vi "RampParaToString_calc.vi"(0 "#Points":u32, 1 "Mode":T1(ring), 3 "RampParameter":dbl[](array[numeric])=[0.0, 30.0, 1.0, 20.0] format="%.2f", 4 "Maximum Allowed Current":dbl=100.0 format="%.2f") -> (5 "Output String":string, 6 "#Points output":u32, 7 "Field Step":dbl=0.5 format="%.2f")   [LabVIEW 2021]
doc: "This Vi extract current field and set the scan continue boolean variable.\n\nThe field step can be either positive or negative.\n\nIf any of the absolute field value exceeds the maximum allowed limit, it will be replaced with the maximum field value itself"
panel:
  out "Field Array List":dbl[](array[numeric])=[0.0, 0.5, 1.0, 1.5, 2.0, 2.5, 3.0, 3.5, 4.0, 4.5, 5.0, 5.5, 6.0, 6.5, 7.0, 7.5, 8.0, 8.5, 9.0, 9.5, 10.0, 10.5, 11.0, 11.5, 12.0, 12.5, 13.0, 13.5, 14.0, 14.5, 15.0, 15.5, 16.0, 16.5, 17.0, 17.5, 18.0, 18.5, 19.0, 19.5, 20.0, 20.5, 21.0, 21.5, 22.0, 22.5, 23.0, 23.5, 24.0, 24.5, 25.0, 25.5, 26.0, 26.5, 27.0, 27.5, 28.0, 28.5, 29.0, 29.5, 30.0, 30.5, 31.0, 31.5, 32.0, 32.5, 33.0, 33.5, 34.0, 34.5, 35.0, 35.5, 36.0, 36.5, 37.0, 37.5, 38.0, 38.5, 39.0, 39.5, 40.0, 40.5, 41.0, 41.5, 42.0, 42.5, 43.0, 43.5, 44.0, 44.5]
  out "Final Field":dbl=45.0 format="%.2f"
  out "Initial Field":dbl format="%.2f"
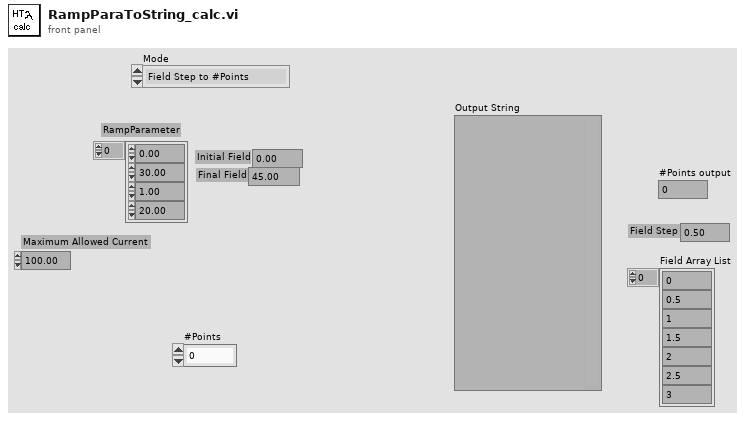
[diagram p1: front panel]
types:
  T1 = enum8{"Field Step to #Points", "#Points to Field Steps"}
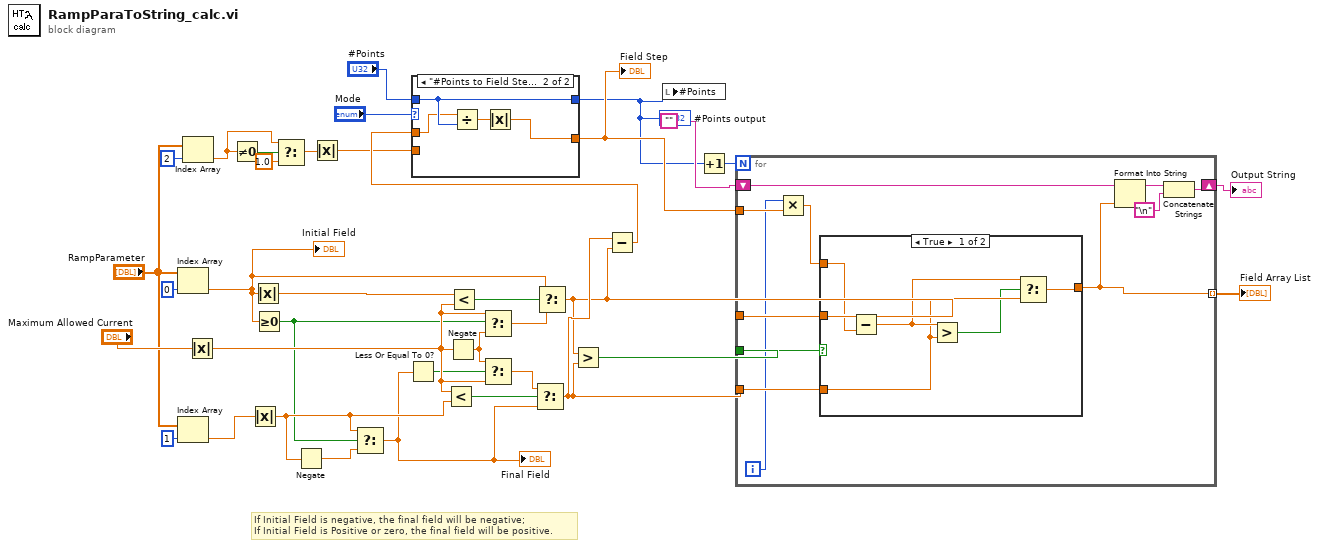
[diagram p0: block diagram]
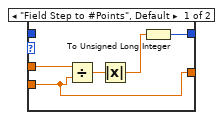
[diagram p2: hidden frame]
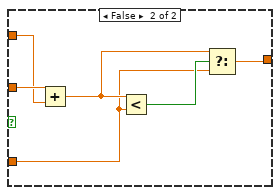
[diagram p3: hidden frame]
diagram:
  # "If Initial Field is negative, the final field will be negative;\nIf Initial Field is Positive or zero, the final field will be positive."
  n1 = Index Array(array="RampParameter", index=0) -> (element=w32:dbl)
  "Initial Field" <- w32
  n2 = Index Array(array="RampParameter", index=1) -> (element=w31:dbl)
  n3 = Index Array(array="RampParameter", index=2) -> (element=w9:dbl)
  n4 = Absolute Value(x="Maximum Allowed Current") -> (abs(x)=w35:dbl)
  n5 = Not Equal To 0?(x=w9) -> (x != 0?=w10:bool)
  n6 = Absolute Value(x=w31) -> (abs(x)=w16:dbl)
  n7 = Absolute Value(x=w32) -> (abs(x)=w36:dbl)
  n8 = Greater Or Equal To 0?(x=w32) -> (x >= 0?=w15:bool)
  n9 = Select(t=w9, s=w10, f=1.0) -> (s? t:f=w4:dbl)
  n10 = Negate(x=w16) -> (-x=w14:dbl)
  n11 = Absolute Value(x=w4) -> (abs(x)=w2:dbl)
  n12 = Select(t=w16, s=w15, f=w14) -> (s? t:f=w13:dbl)
  "Final Field" <- w13
  n13 = Less Or Equal To 0?(x=w13) -> (x <= 0?=w25:bool)
  n14 = Less?(x=w35, y=w16) -> (x < y?=w27:bool)
  n15 = Negate(x=w35) -> (-x=w24:dbl)
  n16 = Less?(x=w36, y=w35) -> (x < y?=w28:bool)
  n17 = Select(t=w35, s=w15, f=w24) -> (s? t:f=w26:dbl)
  n18 = Select(t=w24, s=w25, f=w35) -> (s? t:f=w23:dbl)
  n19 = Select(t=w23, s=w27, f=w13) -> (s? t:f=w22:dbl)
  n20 = Select(t=w32, s=w28, f=w26) -> (s? t:f=w21:dbl)
  n21 = Greater?(x=w21, y=w22) -> (0:w29:bool)
  n22 = Subtract(x=w22, y=w21) -> (x-y=w3:dbl)
  n23 = case shown="\"#Points to Field Steps\"" "Mode" {
    tunnel: w3 -> [w40 w42]
    tunnel: "#Points" -> [_ w44]
    tunnel: [w38 w44] -> w1
    tunnel: [w37 w43] -> w5
    tunnel: w2 -> [w37 _]
    frame "Field Step to #Points", Default {
      n24 = Divide(x=w40, y=w37) -> (x/y=w41:dbl)
      n25 = Absolute Value(x=w41) -> (abs(x)=w39:dbl)
      n26 = To Unsigned Long Integer(number=w39) -> (unsigned 32bit integer=w38:u32)
    }
    frame "#Points to Field Steps" {
      n27 = Divide(x=w42, y=w44) -> (x/y=w45:dbl)
      n28 = Absolute Value(x=w45) -> (abs(x)=w43:dbl)
    }
  }
  "Field Step" <- w5
  "#Points output" <- w1
  n29 = local write "#Points"(w1) -> ()
  n30 = Increment(x=w1) -> (x+1=w17:u32)
  n31 = for {
    N: w17 -> [_]
    tunnel: w29 -> [w56]
    tunnel: w5 -> [w55]
    tunnel: w21 -> [w54]
    tunnel: w22 -> [w53]
    tunnel: [w50] -> w20 mode=indexing
    shift-right: [w46] -> w19
    shift-left: "" -> [w48]
    i -> [w51]
    n32 = Multiply(x=w51, y=w55) -> (x*y=w52:dbl)
    n33 = case shown="True" w56 {
      tunnel: w54 -> [w62 w68]
      tunnel: w53 -> [w58 w64]
      tunnel: w52 -> [w61 w67]
      tunnel: [w60 w63] -> w50
      frame True {
        n34 = Subtract(x=w62, y=w61) -> (x-y=w59:dbl)
        n35 = Greater?(x=w59, y=w58) -> (0:w57:bool)
        n36 = Select(t=w59, s=w57, f=w58) -> (s? t:f=w60:dbl)
      }
      frame False {
        n37 = Add(x=w68, y=w67) -> (x+y=w66:dbl)
        n38 = Less?(x=w66, y=w64) -> (x < y?=w65:bool)
        n39 = Select(t=w66, s=w65, f=w64) -> (s? t:f=w63:dbl)
      }
    }
    n40 = Format Into String(initial string=w48, w50) -> (resulting string=w47:string)  [unwired: 2 in, 1 out]
    n41 = Concatenate Strings(w47, "\n") -> (w46:string)
  }
  "Field Array List" <- w20
  "Output String" <- w19
